vi "channel count.vi"(11 "?":T1(array[cluster]) {"Terminal Configuration" items=["default"=-1, "RSE"=10083, "NRSE"=10078, "Differential"=10106, "Pseudodifferential"=12529]}) -> (3 "Array - Numeric":dbl[](array[numeric]))   [LabVIEW 2024]
panel:
  out "channel text":string
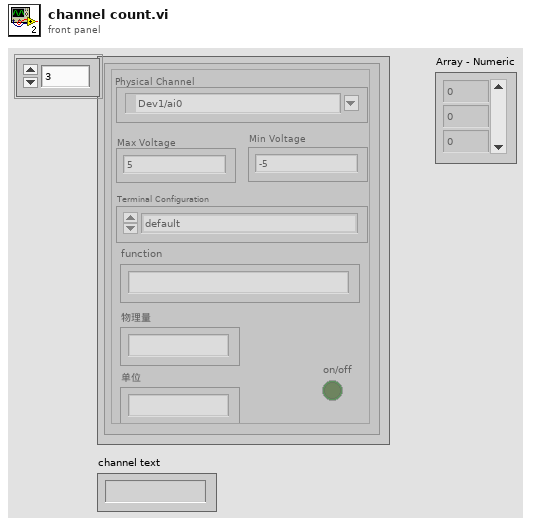
[diagram p1: front panel]
types:
  T1 = cluster{"Terminal Configuration":i32, "Min Voltage":dbl, "Physical Channel":tag, "Max Voltage":dbl, "function":string, "on/off":bool, "物理量":string, "单位":string}[]
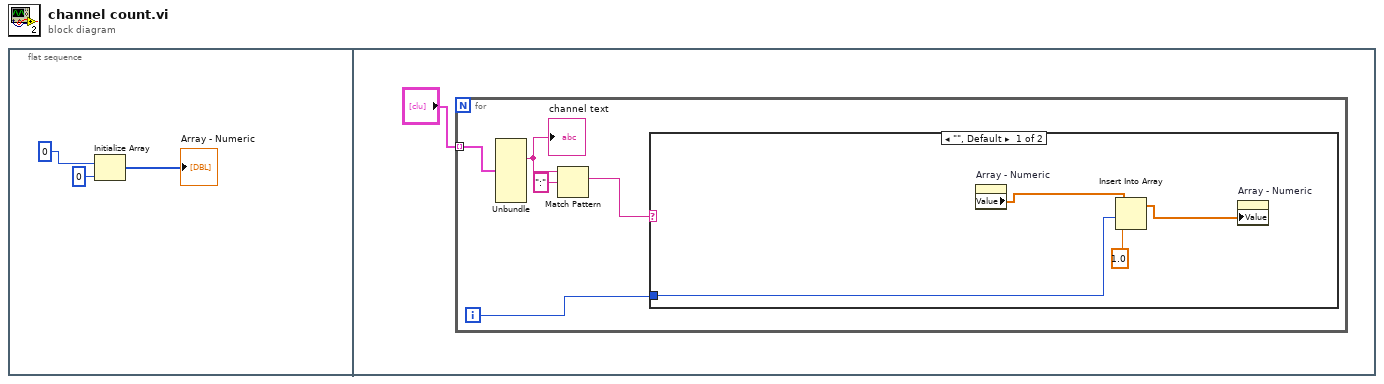
[diagram p0: block diagram]
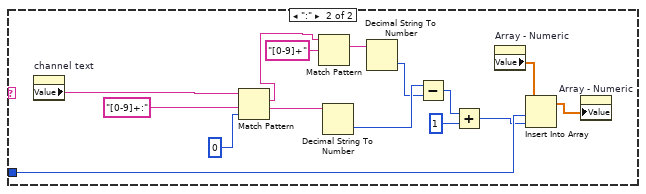
[diagram p2: hidden frame]
diagram:
  n1 = flat-sequence {
    frame #0 {
      n2 = Initialize Array(0, 0 ("dimension size")) -> (→"Array - Numeric":i32[])
    }
    frame #1 {
      n3 = for {
        tunnel: "?" -> [w9] mode=indexing
        i -> [w5]
        n4 = Unbundle(w9) -> ("Physical Channel"=w6:tag)  [unwired: 7 out]
        "channel text" <- w6
        n5 = Match Pattern(string=w6, regular expression=":") -> (match substring=w7:string)  [unwired: 1 in, 3 out]
        n6 = case shown="\"\", Default" w7 {
          tunnel: w5 -> [w13 w16]
          frame "", Default {
            n7 = property on="Array - Numeric" class="Arr (strict)"() -> ("Value"=w11:dbl[])  [unwired: 2 in, 2 out]
            n8 = Insert Into Array(array=w11, index=w13, new element=1.0 ("new element/subarray")) -> (w10:dbl[])
            n9 = property on="Array - Numeric" class="Arr (strict)"("Value"=w10) -> ()  [unwired: 2 in, 2 out]
          }
          frame ":" {
            n10 = property on="channel text" class="Str"() -> ("Value"=w23:string)  [unwired: 2 in, 2 out]
            n11 = Match Pattern(string=w23, regular expression="[0-9]+:", offset (0)=0) -> (match substring=w22:string, after substring=w28:string)  [unwired: 2 out]
            n12 = Match Pattern(string=w22, regular expression="[0-9]+") -> (match substring=w27:string)  [unwired: 1 in, 3 out]
            n13 = Decimal String To Number(string=w28) -> (number=w21:i32)  [unwired: 2 in, 1 out]
            n14 = Decimal String To Number(string=w27) -> (number=w20:i32)  [unwired: 2 in, 1 out]
            n15 = Subtract(x=w21, y=w20) -> (x-y=w19:i32)
            n16 = Add(x=w19, y=1) -> (x+y=w15:i32)
            n17 = property on="Array - Numeric" class="Arr (strict)"() -> ("Value"=w17:dbl[])  [unwired: 2 in, 2 out]
            n18 = Insert Into Array(array=w17, index=w16, new element=w15) -> (w14:dbl[])
            n19 = property on="Array - Numeric" class="Arr (strict)"("Value"=w14) -> ()  [unwired: 2 in, 2 out]
          }
        }
      }
    }
  }
